vi "Example_SubDevice.vi"() -> ()   [LabVIEW 2019, in "maxonEPOS.lvlib"]
doc: "Example how to do a velocity movement. Before starts this example the device must be tuned and the parameter settings must be correct.\nThe example shows:\n - how to initialise and close an interface (e.g. RS232)\n - start of a velocity movement with correct operation mode\n - wait until the target velocity is reached (e.g. 5 seconds)"
uses:
  maxonEPOS.lvlib
panel:
  in  "communication settings subdevice":T1={"deviceName"="EPOS4", "protocolStackName"="CANopen", "baudrate"=1000000}
  in  "nodeId subdevice":u16=2
  in  "timeout subdevice":u32=1000
  in  "velocity profile subdevice":T2={"profileAcceleration"=10000, "profileDeceleration"=10000}
  in  "targetVelocity subdevice":i32=300
  in  "timeout device":u32=1000
  in  "velocity profile device":T2={"profileAcceleration"=10000, "profileDeceleration"=10000}
  in  "communication settings device":T3={"deviceName"="EPOS2", "protocolStackName"="MAXON SERIAL V2", "interfaceName"="USB", "portName"="USB0", "baudrate"=1000000, "timeout"=500}
  in  "milliseconds to wait":u32=5000
  in  "targetVelocity device":i32=300
  in  "nodeId device":u16=1
  # "Device"
  # "Subdevice"
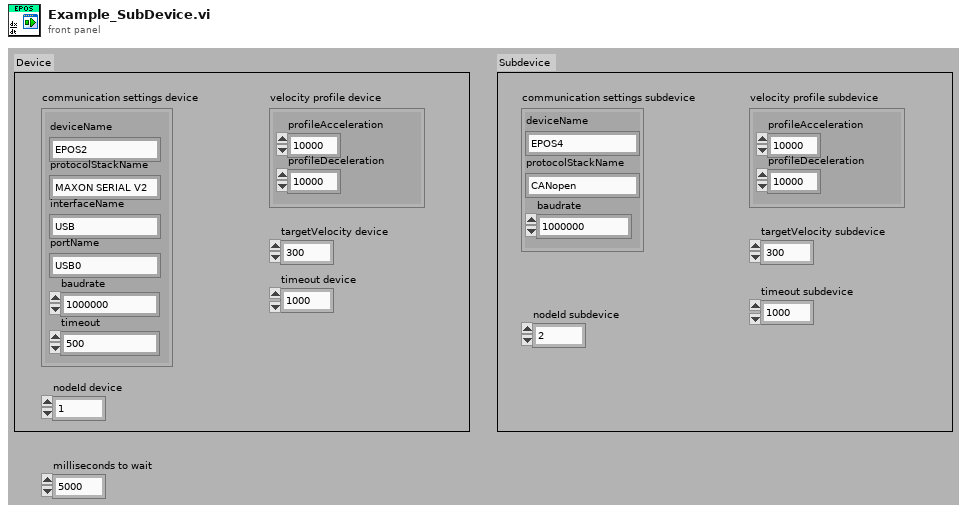
[diagram p1: front panel]
types:
  T1 = cluster{"deviceName":string, "protocolStackName":string, "baudrate":u32}
  T2 = cluster{"profileAcceleration":u32, "profileDeceleration":u32}
  T3 = cluster{"deviceName":string, "protocolStackName":string, "interfaceName":string, "portName":string, "baudrate":u32, "timeout":u32}
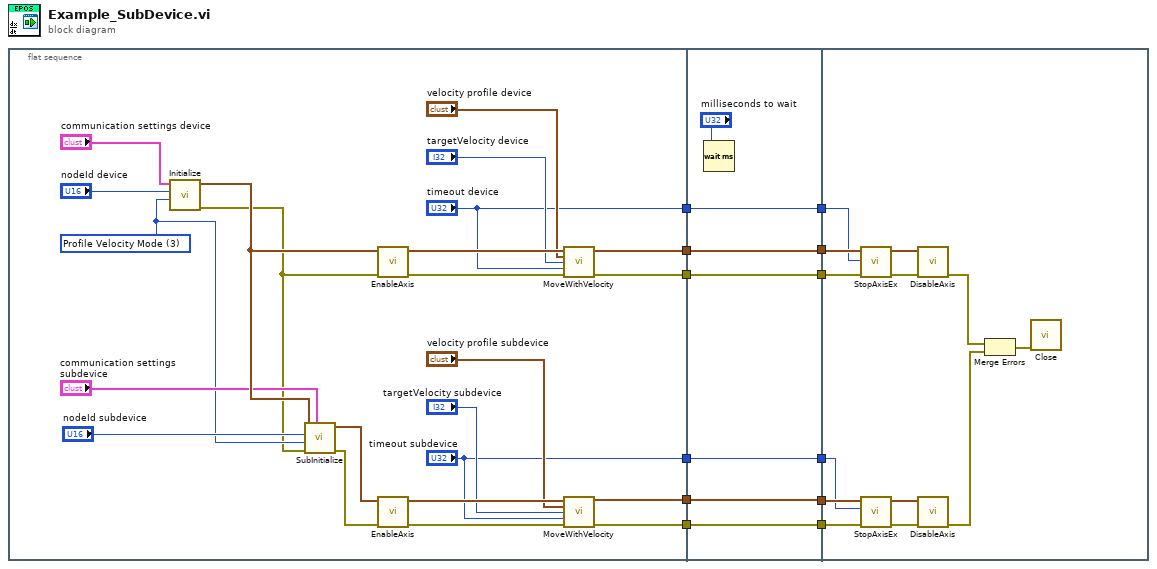
[diagram p0: block diagram]
diagram:
  n1 = flat-sequence {
    tunnel: [w16] -> w11
    tunnel: [w31] -> w9
    tunnel: ["timeout device"] -> w8
    tunnel: [w17] -> w5
    tunnel: [w15] -> w3
    tunnel: ["timeout subdevice"] -> w2
    tunnel: [w41] -> w12
    tunnel: w11 -> [w41]
    tunnel: [w40] -> w10
    tunnel: w9 -> [w40]
    tunnel: w8 -> [w39]
    tunnel: [w39] -> w7
    tunnel: [w38] -> w6
    tunnel: w5 -> [w38]
    tunnel: [w37] -> w4
    tunnel: w3 -> [w37]
    tunnel: w2 -> [w36]
    tunnel: [w36] -> w1
    tunnel: w12 -> [w55]
    tunnel: w10 -> [w53]
    tunnel: w7 -> [w51]
    tunnel: w6 -> [w50]
    tunnel: w4 -> [w45]
    tunnel: w1 -> [w43]
    frame #0 {
      w18 = i8 3 items=["Profile Position Mode"=1, "Profile Velocity Mode"=3, "Homing Mode"=6, "Interpolated Position Mode"=7, "Position Mode"=-1, "Velocity Mode"=-2, "Current Mode"=-3, "Master Encoder Mode"=-5, "Step Direction Mode"=-6] ("modes of operations")
      n2 = call "Initialize.vi"("modes of operations"=w18, "nodeId"="nodeId device", "communication settings in"="communication settings device") -> ("error out"=w13:errorcluster, "axis out"=w21:cluster{"keyHandle":u32, "nodeId":u16})  [unwired: 7 in]
      n3 = call "SubInitialize.vi"("communication settings"="communication settings subdevice", "error in (no error)"=w13, "modes of operations"=w18, "nodeId"="nodeId subdevice", "axis in"=w21) -> ("error out"=w22:errorcluster, "axis out"=w23:cluster{"keyHandle":u32, "nodeId":u16})  [unwired: 5 in]
      n4 = call "EnableAxis.vi"("error in (no error)"=w13, "axis in"=w21) -> ("error out"=w33:errorcluster, "axis out"=w32:cluster{"keyHandle":u32, "nodeId":u16})  [unwired: 4 in]
      n5 = call "EnableAxis.vi"("error in (no error)"=w22, "axis in"=w23) -> ("error out"=w27:errorcluster, "axis out"=w26:cluster{"keyHandle":u32, "nodeId":u16})  [unwired: 4 in]
      n6 = call "MoveWithVelocity.vi"("axis in"=w32, "velocity profile"="velocity profile device", "targetVelocity"="targetVelocity device", "timeout"="timeout device", "error in (no error)"=w33) -> ("axis out"=w31:cluster{"keyHandle":u32, "nodeId":u16}, "error out"=w16:errorcluster)  [unwired: 9 in]
      n7 = call "MoveWithVelocity.vi"("axis in"=w26, "velocity profile"="velocity profile subdevice", "targetVelocity"="targetVelocity subdevice", "timeout"="timeout subdevice", "error in (no error)"=w27) -> ("axis out"=w17:cluster{"keyHandle":u32, "nodeId":u16}, "error out"=w15:errorcluster)  [unwired: 9 in]
    }
    frame #1 {
      n8 = Wait (ms)(milliseconds to wait="milliseconds to wait") -> ()  [unwired: 1 out]
    }
    frame #2 {
      n9 = call "StopAxisEx.vi"("error in (no error)"=w55, "timeout"=w51, "axis in"=w53) -> ("error out"=w54:errorcluster, "axis out"=w52:cluster{"keyHandle":u32, "nodeId":u16})  [unwired: 3 in]
      n10 = call "StopAxisEx.vi"("error in (no error)"=w45, "timeout"=w43, "axis in"=w50) -> ("error out"=w44:errorcluster, "axis out"=w49:cluster{"keyHandle":u32, "nodeId":u16})  [unwired: 3 in]
      n11 = call "DisableAxis.vi"("error in (no error)"=w54, "axis in"=w52) -> ("error out"=w47:errorcluster)  [unwired: 4 in, 1 out]
      n12 = call "DisableAxis.vi"("error in (no error)"=w44, "axis in"=w49) -> ("error out"=w48:errorcluster)  [unwired: 4 in, 1 out]
      n13 = Merge Errors(w47, w48) -> (w46:errorcluster)
      n14 = call "Close.vi"("error in (no error)"=w46) -> ()  [unwired: 10 in, 1 out]
    }
  }
